vi "pid 제어.vi"() -> ()   [LabVIEW 2016]
uses:
  <vilib>/Platform/TimedLoop/XDataNode/timing_clust.ctl
  <vilib>/Platform/TimedLoop/XDataNode/nitl_modes.ctl
  <vilib>/Platform/TimedLoop/XDataNode/wakeup.ctl
  <vilib>/addons/control/pid/pid.llb/PID (DBL).vi
  <vilib>/addons/control/pid/pid.llb/PID Lead-Lag (DBL).vi
  <vilib>/Platform/TimedLoop/XDataNode/XDataNode.xnode
  <vilib>/express/express arith-compare/Formula/XNode/ExpressFormulaBlockNode.xnode
  <vilib>/addons/control/pid/NI_PID_pid.lvlib
  <vilib>/Platform/TimedLoop/XDataNode/XDNodeRunTimeDep.lvlib
panel:
  in  "V0":dbl
  out "brake":i16
  in  "S":dbl=0.5 format="%#_13g"
  in  "V":dbl=4.0 format="%#_13g"
  in  "정지":bool
  out "PV Setpoint Output":cluster{"initial PV":dbl, "setpoint":dbl}(graph)={"initial PV"=0.18693112703744846, "setpoint"=0.0}
  in  "PID gains":T1={"proportional gain (Kc)"=1.0, "integral time (Ti, min)"=0.01, "derivative time (Td, min)"=0.0} caption="PID 게인" {"derivative time (Td, min)" format="%#.6g"; "integral time (Ti, min)" format="%#.6g"; "proportional gain (Kc)" format="%#.6g"}
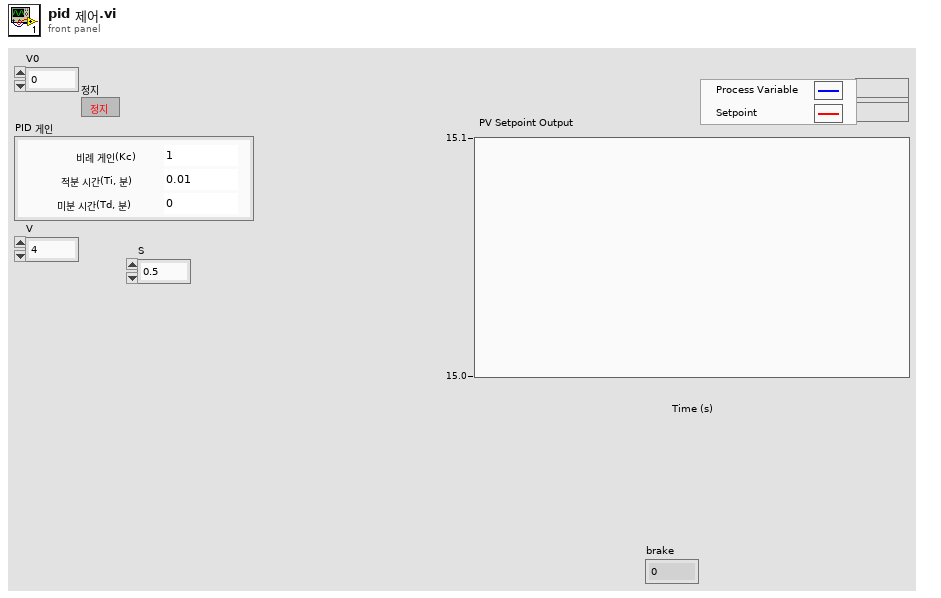
[diagram p1: front panel]
types:
  T1 = cluster{"proportional gain (Kc)":dbl, "integral time (Ti, min)":dbl, "derivative time (Td, min)":dbl}
  T2 = typedef "XDNodeRunTimeDep.lvlib/timing_clust.ctl" = cluster{"Expected End [f-1]":u64, "Actual End [f-1]":u64, "Finished Late? [f-1]":bool, "Expected End [i-1]":u64, "Actual End [i-1]":u64, "Finished Late? [i-1]":bool, "Expected Start [i]":u64, "Actual Start [i]":u64, "Expected Start [f]":u64, "Actual Start [f]":u64, "Source Name":string, "Structure Name":string, "Period":i64, "Deadline":i64, "Offset":i64, "Start":i64, "Priority":i32, "Timeout":i32, "Mode":T3, "Wakeup Reason":T4, "Error":errorcluster, "Source Type":string, "Secondary Source Type":string, "Global End Time":u64, "Global Start Time":u64, "Frame Duration":u64, "Iteration Duration":u64, "Assigned CPU":i32, "I/O Scan Engine Mode":u32}
  T3 = typedef "XDNodeRunTimeDep.lvlib/nitl_modes.ctl" = enum32{"No Change", "Process missed periods, maintain original phase", "Discard missed periods, maintain original phase", "Process missed periods, ignore original phase", "Discard missed periods, ignore original phase"}
  T4 = typedef "XDNodeRunTimeDep.lvlib/wakeup.ctl" = enum32{"Normal", "Aborted", "Asynchronous wakeup", "Timing source error", "Timed loop error", "Timeout"}
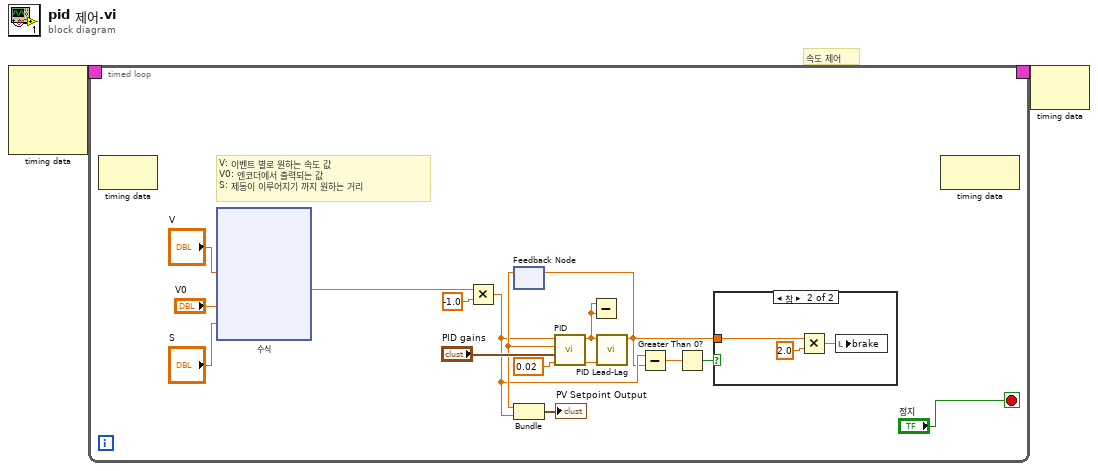
[diagram p0: block diagram]
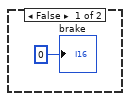
[diagram p2: hidden frame]
diagram:
  # "속도 제어"
  n1 = node-c288() -> (w2:T2)  [unwired: 4 in]
  n2 = timed-loop {
    timing: w2 -> [_]
    timing-out: [_] -> w1
    stop <- "정지" stop-if-true
    # "V: 이벤트 별로 원하는 속도 값\nV0: 엔코더에서 출력되는 값\nS: 제동이 이루어지기 까지 원하는 거리"
    n3 = node-c288() -> ()  [unwired: 1 in, 1 out]
    n4 = xnode "수식"("V"="V", "V0"="V0", "S"="S") -> ("결과"=w8:dbl)  [unwired: 1 in, 1 out]
    n5 = Multiply(x=w8, y=-1.0) -> (x*y=w6:dbl)
    n6 = feedback #1() -> (w15:dbl)  [unwired: 1 in]
    n7 = Bundle("output"=w15, w6) -> (→"PV Setpoint Output":cluster{"output":dbl, dbl})  [unwired: 1 in]
    n8 = call-poly <vilib>:"PID.vi"("dt (s)"=0.02, "PID gains"="PID gains", "process variable"=w15, "setpoint"=w6) -> ("dt out (s)"=w13:dbl, "output"=w12:dbl)  [unwired: 6 in]
    n9 = Subtract(x=w12, y=w12) -> ()  [unwired: 1 out]
    n10 = call-poly <vilib>:"PID Lead-Lag.vi"("dt (s)"=w13, "input"=w12) -> ("output"=w5:dbl)  [unwired: 6 in, 1 out]
    n11 = feedback-in #1(w5) -> ()
    n12 = Subtract(x=w6, y=w5) -> (x-y=w4:dbl)
    n13 = Greater Than 0?(x=w4) -> (x > 0?=w7:bool)
    n14 = case shown="참" w7 {
      tunnel: w5 -> [_ w34]
      frame False {
        "brake" <- i16 0 ("brake")
      }
      frame True {
        n15 = Multiply(x=w34, y=2.0) -> (x*y=w33:dbl)
        n16 = local write "brake"(w33) -> ()
      }
    }
    n17 = node-c288() -> ()  [unwired: 1 in, 1 out]
  }
  n18 = node-c288(w1) -> ()  [unwired: 1 out]
